vi "FL_Collect_Timings_Data.vi"(0 "Control":refnum<queue>, 1 "Progress Bar Dialog in":refnum<class "Progress Bar Dialog.lvclass">, 5 "States":refnum<notifier>, 7 "Calibration buffer length, samples":i32=1000, 9 "Reset":bool, 11 "error in (no error)":errorcluster, 12 "Data in":T2) -> (4 "Calibration HW timings":u32[](array[numeric]), 6 "Calibration SW timings":dbl[](array[numeric]), 10 "Done":bool, 15 "error out":errorcluster)   [LabVIEW 2018, in "Tracker.lvlib"]
uses:
  Tracker.lvlib
  Controls/CTL_Control_States.ctl
  Controls/CTL_States_cluster.ctl
  Controls/CTL_Animal_Coordinates_and_Speed.ctl
  <vilib>/ProgressBar/Progress Bar Dialog.lvclass
  3ae59c51-e7d8-44f4-b3ac-aa476e3ff834.vi
  5999c7f2-9bf1-42b8-9b28-a6f12208fd2c.vi
  3ae59c51-e7d8-44f4-b3ac-aa476e3ff834.vi/ae92b8c7-68f3-4ff2-b52d-53f615c3f079.vi
  5999c7f2-9bf1-42b8-9b28-a6f12208fd2c.vi/09e640d7-c180-4347-b969-27d18d988134.vi
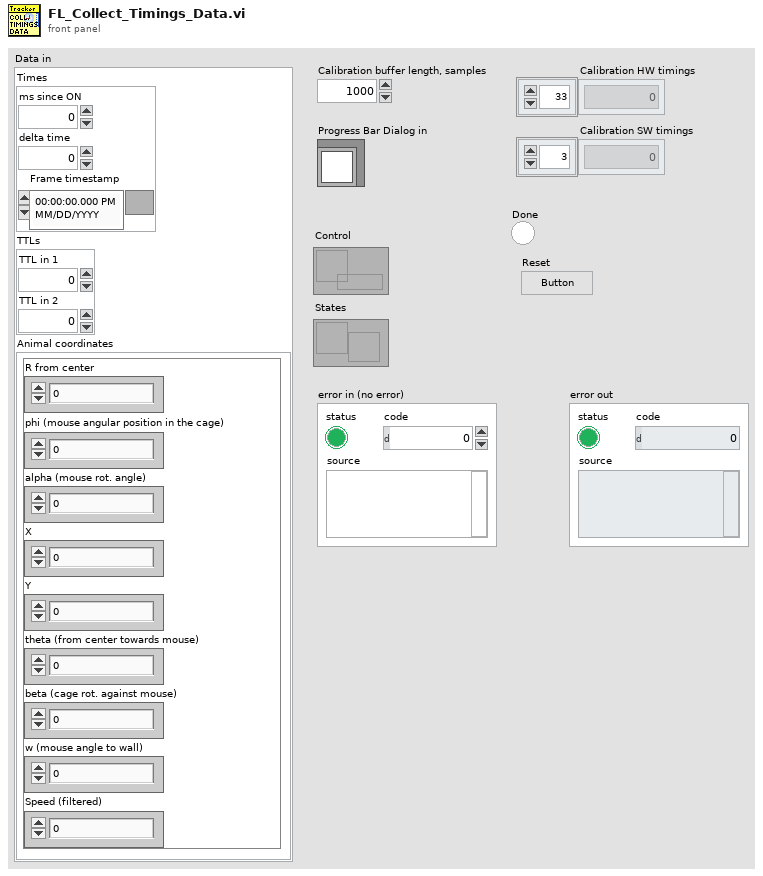
[diagram p1: front panel]
types:
  T1 = typedef "Tracker.lvlib/CTL_Animal_Coordinates_and_Speed.ctl" = cluster{"R from center":dbl, "phi (mouse angular position in the cage)":dbl, "alpha (mouse rot. angle)":sgl, "X":dbl, "Y":dbl, "theta (from center towards mouse)":dbl, "beta (cage rot. against mouse)":sgl, "w (mouse angle to wall)":dbl, "Speed (filtered)":dbl}
  T2 = cluster{"Times":cluster{"ms since ON":u32, "delta time":u32, "Frame timestamp":timestamp}, "TTLs":cluster{"TTL in 1":i16, "TTL in 2":i16}, "Animal coordinates":T1}
  T3 = cluster{"ms since ON":u32, "delta time":u32, "Frame timestamp":timestamp}
  T4 = typedef "Tracker.lvlib/CTL_Control_States.ctl" = enum16{"SW Init", "HW Init", "Close App", "Update port info (Init OK)", "Unlock UI (init OK)", "Save HW Settings", "Re-check HW (init failed)", "Configure port(s)", "Switch to Offline mode", "Zones layout update", "Set I/O config", "Reset stimulus", "Reset zones", "Play Start", "Play Stop", "Upd. FPS", "Upd. trace length", "Cage and recording settings", "Update filter", "Timings calibration start", "Timings calibration finish", "Dispension calibration", "Save all settings"}
  T5 = typedef "Tracker.lvlib/CTL_States_cluster.ctl" = cluster{"Acq. is ON":bool, "Playing loaded":bool, "Recording now":bool, "Has been recorded":bool, "Data saved":bool, "Data loaded":bool, "Calibration mode":bool, "Offline mode":bool, "Stop and Exit":bool}
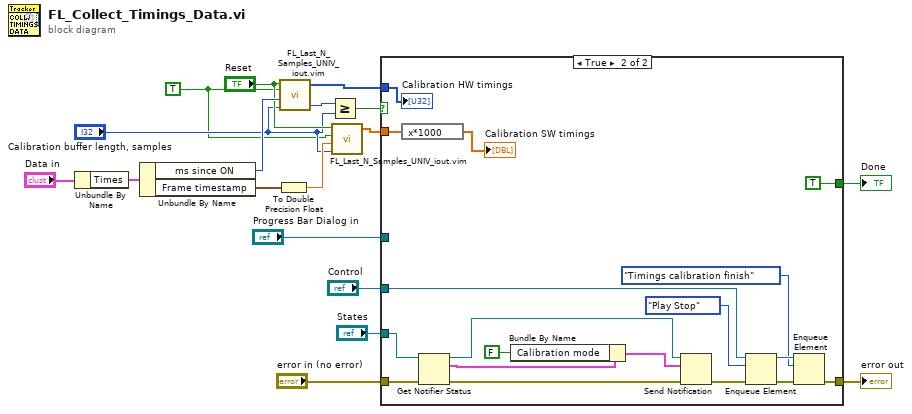
[diagram p0: block diagram]
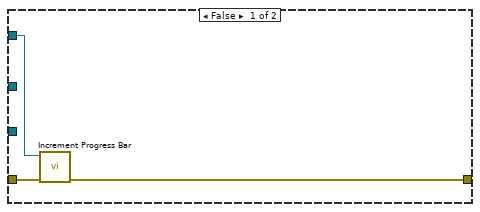
[diagram p2: hidden frame]
diagram:
  w1 = TRUE ("Flip buffer output (F)")
  n1 = Unbundle By Name("Data in") -> ("Times"=w7:T3)
  n2 = Unbundle By Name(w7) -> ("ms since ON"=w8:u32, "Frame timestamp"=w9:timestamp)
  n3 = To Double Precision Float(number=w9) -> (double precision float=w18:dbl)
  n4 = call "FL_Last_N_Samples_UNIV_iout.vim"("Buffer length, samples"="Calibration buffer length, samples", "Input sample"=w8, "Flip buffer output (F)"=w1, "Reset buffer"="Reset") -> ("Current buffer length, samples"=w10:i32, "Output Array"=w12:u32[])  [unwired: 1 out]
  n5 = Greater Or Equal?(x=w10, y="Calibration buffer length, samples") -> (x >= y?=w11:bool)
  n6 = call "FL_Last_N_Samples_UNIV_iout.vim"("Buffer length, samples"="Calibration buffer length, samples", "Input sample"=w18, "Flip buffer output (F)"=w1, "Reset buffer"="Reset") -> ("Output Array"=w13:dbl[])  [unwired: 2 out]
  n7 = case shown="True" w11 {
    tunnel: w12 -> [_ w29]
    tunnel: w13 -> [_ w39]
    tunnel: "error in (no error)" -> [w21 w27]
    tunnel: [w20 w31] -> w15
    tunnel: "States" -> [_ w25]
    tunnel: "Control" -> [_ w35]
    tunnel: "Progress Bar Dialog in" -> [w19 _]
    tunnel: [_ TRUE] -> w2
    frame False {
      n8 = call <vilib>:"Increment Progress Bar.vi"("error in (no error)"=w21, "Progress Bar Dialog in"=w19) -> ("error out"=w20:errorcluster)  [unwired: 7 in, 2 out]
    }
    frame True {
      n9 = expression code="x*1000"(w39) -> (→"Calibration SW timings":dbl[])
      n10 = Get Notifier Status(notifier=w25, error in (no error)=w27) -> (notifier out=w24:refnum<notifier>, current notification=w23:T5, error out=w26:errorcluster)  [unwired: 2 out]
      n11 = Bundle By Name(cluster=w23, "Calibration mode"=FALSE) -> (w38:T5)
      n12 = Send Notification(notification=w38, notifier=w24, error in (no error)=w26) -> (error out=w36:errorcluster)  [unwired: 1 out]
      n13 = Enqueue Element(queue=w35, element=CTL_Control_States."Play Stop", error in (no error)=w36) -> (queue out=w32:refnum<queue>, error out=w33:errorcluster)  [unwired: 1 in, 1 out]
      n14 = Enqueue Element(queue=w32, element=CTL_Control_States."Timings calibration finish", error in (no error)=w33) -> (error out=w31:errorcluster)  [unwired: 1 in, 2 out]
      "Calibration HW timings" <- w29
    }
  }
  "error out" <- w15
  "Done" <- w2
